vi "Test Passing.vi"(8 "error in (no error)":errorcluster, 11 "LUnit Setup Error in":refnum<class "LUnit Tear Down Error.lvclass">) -> (0 "error out":errorcluster, 3 "LUnit Setup Error out":refnum<class "LUnit Tear Down Error.lvclass">)   [LabVIEW 2020, in "LUnit Tear Down Error.lvclass"]
uses:
  LUnit Tear Down Error.lvclass
  C:/Program Files (x86)/National Instruments/LabVIEW 2020/vi.lib/Asteme/LUnit/Test Case.lvclass
  <vilib>/Asteme/LUnit/Test Case.lvclass/Test Case.ctl
  <vilib>/Asteme/LUnit/LUnit Assertion Result.lvclass/LUnit Assertion Result.ctl
  <vilib>/Asteme/LUnit/Add test result.vi
  <vilib>/Asteme/LUnit/LUnit Write Passed.vi
  <vilib>/Asteme/LUnit/LUnit Write Message.vi
  <vilib>/Asteme/LUnit/LUnit Write Description.vi
  <vilib>/Asteme/LUnit/Set Assertion Type.vi
  <vilib>/Asteme/LUnit/LUnit Write Assertion Type.vi
  <vilib>/Asteme/LUnit/Assertion Result/LUnit Get Test Name.vi
  <vilib>/Asteme/LUnit/LUnit Get Test Case.vi
  <vilib>/Asteme/LUnit/LUnit Assertion Result.lvclass
  <vilib>/Asteme/LUnit/Test Case.lvclass
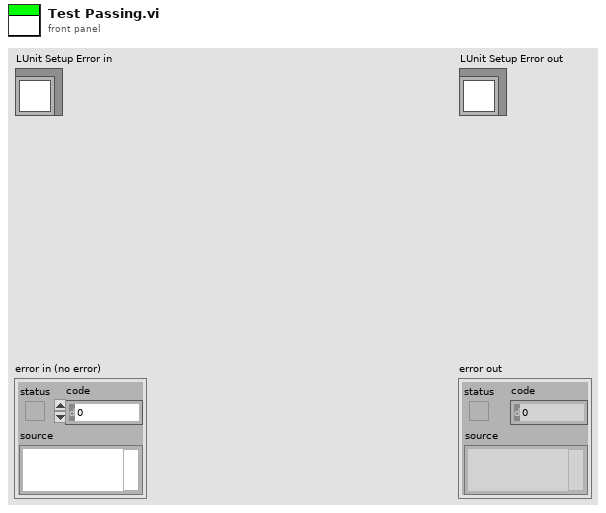
[diagram p1: front panel]
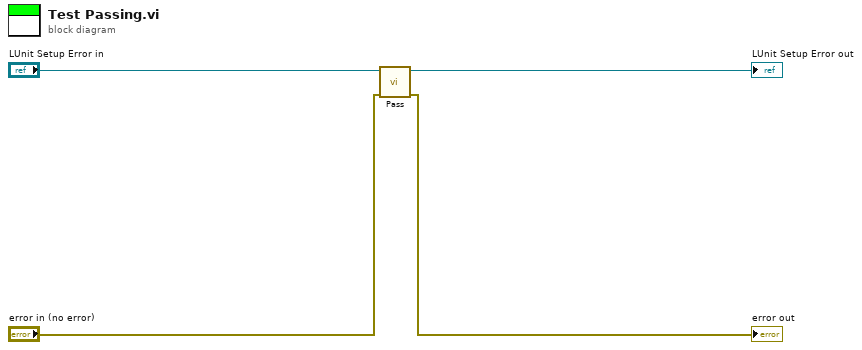
[diagram p0: block diagram]
diagram:
  n1 = call <vilib>:"Pass.vi"("error in (no error)"="error in (no error)", "Test Case In"="LUnit Setup Error in") -> ("error out"=→"error out":errorcluster, "Test Case Out"=→"LUnit Setup Error out":refnum<class "LUnit Tear Down Error.lvclass">)  [unwired: 8 in]
